vi "Tosca-Init Masker Stimulus.vi"(0 "task in":refnum<k21>, 7 "Channel":refnum<class "Channel.lvclass">, 11 "error in (no error)":errorcluster, 12 "Sampling rate (Hz)":dbl, 13 "Npts":i32) -> (4 "task out":refnum<k21>, 8 "Channel out":refnum<class "Channel.lvclass">, 14 "Ramp (ms)":dbl, 15 "error out":errorcluster)   [LabVIEW 2020]
uses:
  epl-vi-lib/Signal Synthesis VIs/4th Generation/Classes/Channel/Channel.lvclass
  epl-vi-lib/Signal Synthesis VIs/4th Generation/Classes/Channel/Channel.lvclass/Channel.ctl
  epl-vi-lib/Signal Synthesis VIs/4th Generation/Classes/Level/Level.lvclass/Level.ctl
  <vilib>/DAQmx/write.llb/DAQmx Write (Analog 1D DBL 1Chan NSamp).vi
  epl-vi-lib/Signal Synthesis VIs/4th Generation/Classes/Channel/Read Level Value.vi
  epl-vi-lib/Signal Synthesis VIs/4th Generation/Classes/Level/Read Level.vi
  Sub VIs/Tosca-Globals.vi
  <vilib>/DAQmx/miscellaneous.llb/DAQmx Fill In Error Info.vi
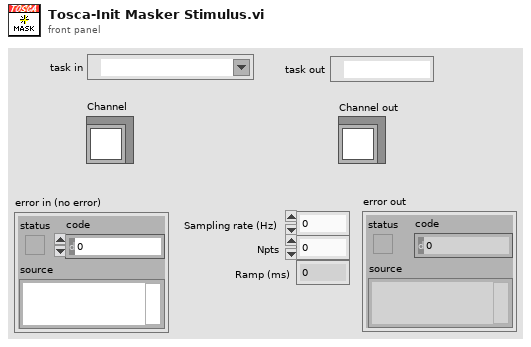
[diagram p1: front panel]
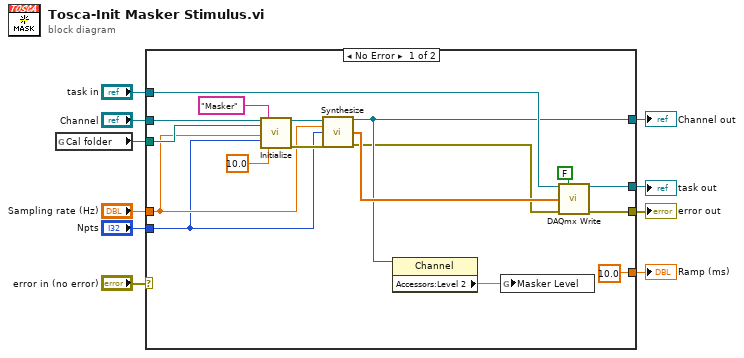
[diagram p0: block diagram]
diagram:
  n1 = global read "Tosca-Globals.vi" "Cal folder"() -> (w2:path)
  n2 = case shown="No Error" "error in (no error)" {
    selector: "error in (no error)" -> [_ w28]
    tunnel: "Npts" -> [w11 _]
    tunnel: "Sampling rate (Hz)" -> [w17 _]
    tunnel: [w14 _] -> w1
    tunnel: [w27 _] -> w8
    tunnel: [w26 w28] -> w7
    tunnel: [10.0 _] -> w5
    tunnel: "task in" -> [w24 _]
    tunnel: "Channel" -> [w23 _]
    tunnel: w2 -> [w22 _]
    frame No Error {
      n3 = call "Initialize.vi"("Channel in"=w23, "Calibration folder"=w22, "Fs (Hz)"=w17, "Npts"=w11, "SigMan Name"="Masker", "Vmax"=10.0) -> ("Channel out"=w19:refnum<class "Channel.lvclass">, "error out"=w18:errorcluster)  [unwired: 12 in]
      n4 = call "Synthesize.vi"("Channel in"=w19, "Fs (Hz)"=w17, "Npts"=w11, "error in (no error)"=w18) -> ("Channel out"=w14:refnum<class "Channel.lvclass">, "Array"=w16:dbl[], "error out"=w13:errorcluster)  [unwired: 8 in, 1 out]
      n5 = property class="Channel"(reference=w14) -> ("Accessors:Level 2"=w12:dbl)  [unwired: 1 in, 2 out]
      n6 = global write "Tosca-Globals.vi" "Masker Level"(w12) -> ()
      n7 = call-poly <vilib>:"DAQmx Write.vi"("task/channels in"=w24, "auto start"=FALSE, "data"=w16, "error in"=w13) -> ("task out"=w27:refnum<k21>, "error out"=w26:errorcluster)  [unwired: 9 in, 1 out]
    }
    frame Error {
    }
  }
  "error out" <- w7
  "task out" <- w8
  "Ramp (ms)" <- w5
  "Channel out" <- w1
